vi "prueba camera control.vi"() -> ()   [LabVIEW 2010]
uses:
  <vilib>/addons/PixeLINK/Low Level Functions/CAMERA_FEATURES.llb/TDPU-CameraFeatures-PixelFormat.ctl
  <vilib>/vision/Image Controls.llb/IMAQ Image.ctl
panel:
  in  "Mostrar?":bool
  out "tiempo (ms)":u32
  out "errorCamera":errorcluster
  out "Image Device OUT":cluster{"Image":T1, "errorImage":errorcluster}
  out "Boolean":bool
  in  "Camera Parameters":T3 {"Pixel Format" items=["PIXEL_FORMAT_MONO8", "PIXEL_FORMAT_MONO16", "PIXEL_FORMAT_YUV422", "PIXEL_FORMAT_BAYER8_GRBG", "PIXEL_FORMAT_BAYER16_GRBG", "PIXEL_FORMAT_RGB24", "PIXEL_FORMAT_RGB48", "PIXEL_FORMAT_BAYER8_RGGB", "PIXEL_FORMAT_BAYER8_GBRG ", "PIXEL_FORMAT_BAYER8_BGGR ", "PIXEL_FORMAT_BAYER16_RGGB ", "PIXEL_FORMAT_BAYER16_GBRG", "PIXEL_FORMAT_BAYER16_BGGR", "PIXEL_FORMAT_RGB32"]}
  in  "Selector":u16(ring) items=["776002034"]
  in  "stop":bool
  in  "Streeam?":bool
  out "Image":T1(plugin-control)
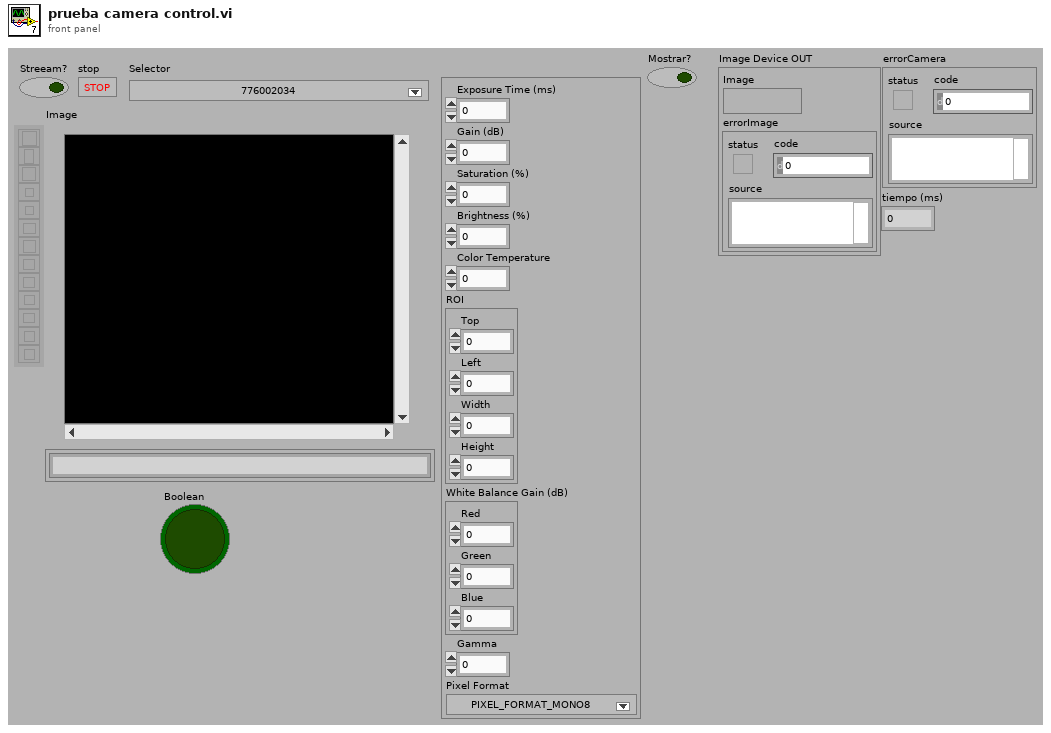
[diagram p1: front panel]
types:
  T1 = typedef "IMAQ Image.ctl" = refnum<image>
  T2 = typedef "TDPU-CameraFeatures-PixelFormat.ctl" = u16
  T3 = cluster{"Exposure Time (ms)":u32, "Gain (dB)":dbl, "Saturation (%)":dbl, "Brightness (%)":dbl, "Color Temperature":dbl, "ROI":cluster{"Top":i32, "Left":i32, "Width":i32, "Height":i32}, "White Balance Gain (dB)":cluster{"Red":dbl, "Green":dbl, "Blue":dbl}, "Gamma":dbl, "Pixel Format":T2}
  T4 = cluster{"hCamera":u32, "Error":errorcluster, "uSerialNumber OUT":u32}
  T5 = typedef "Image Type" = u32
  T6 = cluster{"hCamera":u32, "Error":errorcluster, "uSerialNumber":u32}
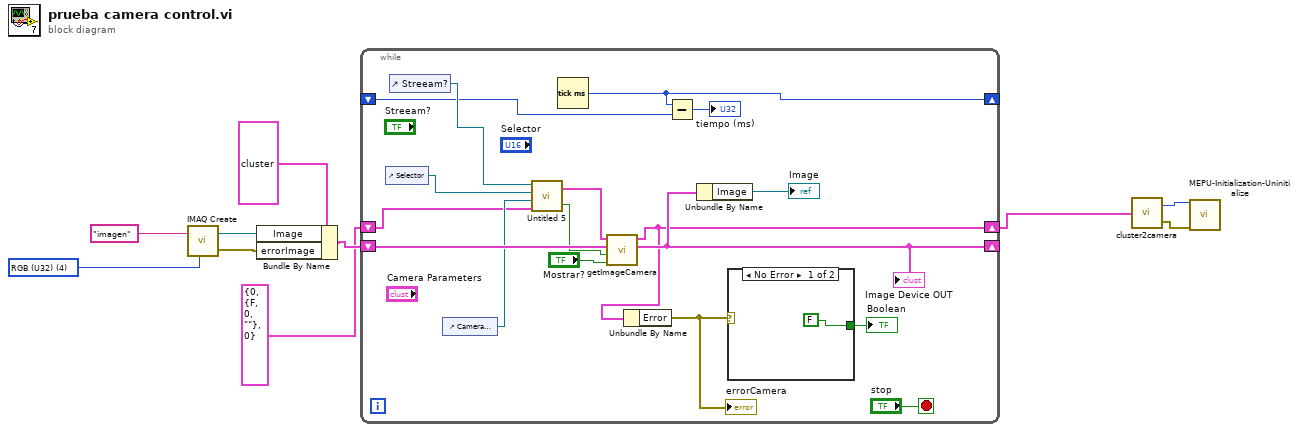
[diagram p0: block diagram]
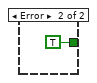
[diagram p2: hidden frame]
diagram:
  w8 = T5 4 items=["Grayscale (U8)", "Grayscale (I16)", "Grayscale (SGL)", "Complex (CSG)", "RGB (U32)", "HSL (U32)", "RGB (U64)", "Grayscale (U16)"] ("Image Type")
  n1 = call "IMAQ Create"("Image Name"="imagen", "Image Type"=w8) -> ("New Image"=w9:T1, "error out"=w10:errorcluster)  [unwired: 3 in]
  n2 = Bundle By Name(cluster=cluster{"Image":T1, "errorImage":errorcluster} {"Image"=refnum, "errorImage"={"status"=FALSE, "code"=0, "source"=""}} ("Image Device IN"), "Image"=w9, "errorImage"=w10) -> (w6:cluster{"Image":T1, "errorImage":errorcluster})
  n3 = while {
    shift-right: [w22] -> _
    shift-left: w6 -> [w25]
    shift-right: [w18] -> w1
    shift-left: T4 {"hCamera"=0, "Error"={"status"=FALSE, "code"=0, "source"=""}, "uSerialNumber OUT"=0} ("Camera Device  IN") -> [w16]
    shift-right: [w14] -> _
    shift-left: _ -> [w13]
    stop <- "stop" stop-if-true
    n4 = control-ref of="Selector"() -> (w24:refnum<vi>)
    n5 = control-ref of="Streeam?"() -> (w19:refnum<vi>)
    n6 = control-ref of="Camera Parameters"() -> (w23:refnum<vi>)
    n7 = call "Untitled 5.vi"("Camera Device  IN"=w16, "Camera Parameters"=w23, "Selector"=w24, "Stream?"=w19) -> ("Stream? OUT"=w17:bool, "Camera Device OUT"=w15:T6)
    n8 = Tick Count (ms)() -> (millisecond timer value=w14:u32)
    n9 = call "getImageCamera.vi"("Mostrar?"="Mostrar?", "Streeam?"=w17, "Image Device IN"=w25, "Camera Device  IN"=w15) -> ("Image Device OUT"=w22:cluster{"Image":T1, "errorImage":errorcluster}, "Camera Device OUT"=w18:T4)  [unwired: 1 in, 1 out]
    "Image Device OUT" <- w22
    n10 = Unbundle By Name(w18) -> ("Error"=w21:errorcluster)
    "errorCamera" <- w21
    n11 = Subtract(x=w14, y=w13) -> (x-y=→"tiempo (ms)":u32)
    n12 = Unbundle By Name(w22) -> ("Image"=→"Image":T1)
    n13 = case shown="No Error" w21 {
      tunnel: [FALSE TRUE] -> w20
      frame No Error {
      }
      frame Error {
      }
    }
    "Boolean" <- w20
  }
  n14 = call "cluster2camera.vi"("Camera Device IN"=w1) -> ("Error OUT"=w3:errorcluster, "hCamera OUT"=w4:u32)  [unwired: 2 in, 1 out]
  n15 = call <vilib>:"MEPU-Initialization-Uninitialize.vi"("hCamera IN"=w4, "Error IN"=w3) -> ()  [unwired: 13 in, 1 out]
